vi "FG Sequence Number.vi"(1 "FG Action (Read)":T1, 2 "Sequence Number in":u16) -> (0 "Sequence Number out":u16)   [LabVIEW 2011]
uses:
  cRIO/Functional Global Variables/Actions for FG's.ctl
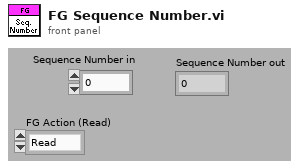
[diagram p1: front panel]
types:
  T1 = typedef "Actions for FG's.ctl" = enum16{"Read", "Write"}
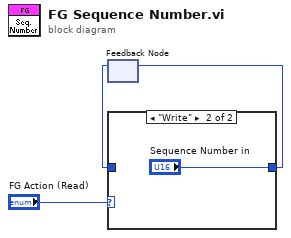
[diagram p0: block diagram]
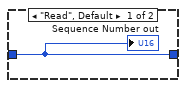
[diagram p2: hidden frame]
diagram:
  n1 = feedback #1() -> (w1:u16)  [unwired: 1 in]
  n2 = case shown="\"Write\"" "FG Action (Read)" {
    tunnel: w1 -> [w4 _]
    tunnel: [w4 "Sequence Number in"] -> w2
    frame "Read", Default {
      "Sequence Number out" <- w4
    }
    frame "Write" {
    }
  }
  n3 = feedback-in #1(w2) -> ()
